vi "Global - Demo Mode Flags.vi"() -> ()   [LabVIEW 2014]
panel:
  in  "System":string
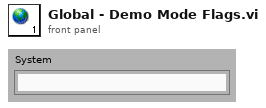
[diagram p1: front panel]
diagram:
